vi "Function.vi"(8 "error in (no error)":errorcluster, 10 "Value":ext, 11 "Two Terminal in":refnum<class "Invert_EXT.lvclass">) -> (0 "error out":errorcluster, 2 "Result":ext, 3 "Two Terminal out":refnum<class "Invert_EXT.lvclass">)   [LabVIEW 2021, in "Invert_EXT.lvclass"]
uses:
  Invert_EXT.lvclass
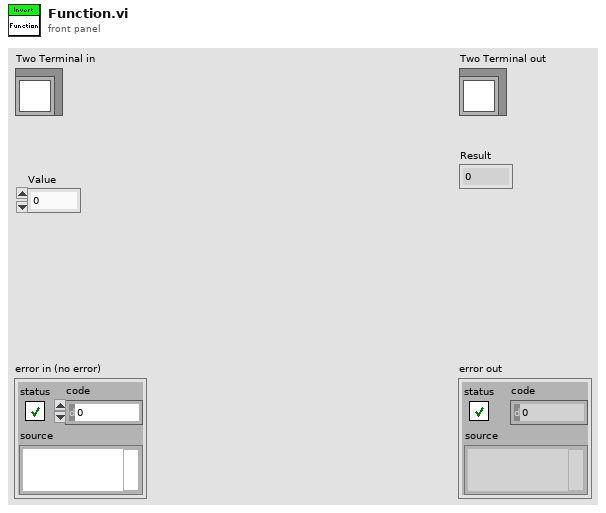
[diagram p1: front panel]
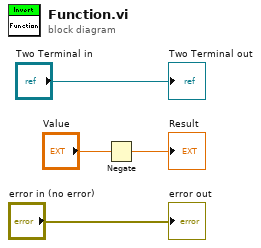
[diagram p0: block diagram]
diagram:
  n1 = Negate(x="Value") -> (-x=→"Result":ext)
  "error out" <- "error in (no error)"
  "Two Terminal out" <- "Two Terminal in"
